vi "parameter error estimate.vi"(8 "covariance":T1, 9 "best fit parameters":dbl[](array[numeric]), 10 "best nonlinear fit":dbl[](array[numeric]), 11 "Y":dbl[](array[numeric])) -> (1 "R-square":dbl, 2 "FWHM":dbl, 3 "Parameters Fit":T2)   [LabVIEW 2023]
uses:
  <vilib>/Analysis/Matrix/Datatypes/RealMatrix.ctl
  <vilib>/Analysis/Matrix/Numeric/Conversions/Array To Matrix - RA2.vi
  <vilib>/Analysis/NI_AALPro.lvlib
  <vilib>/Analysis/Matrix/NI_Matrix.lvlib
panel:
  out "Correlation Matrix":T1
  out "Error":dbl[](array[numeric])
  out "RMSE":dbl
  out "SSE":dbl
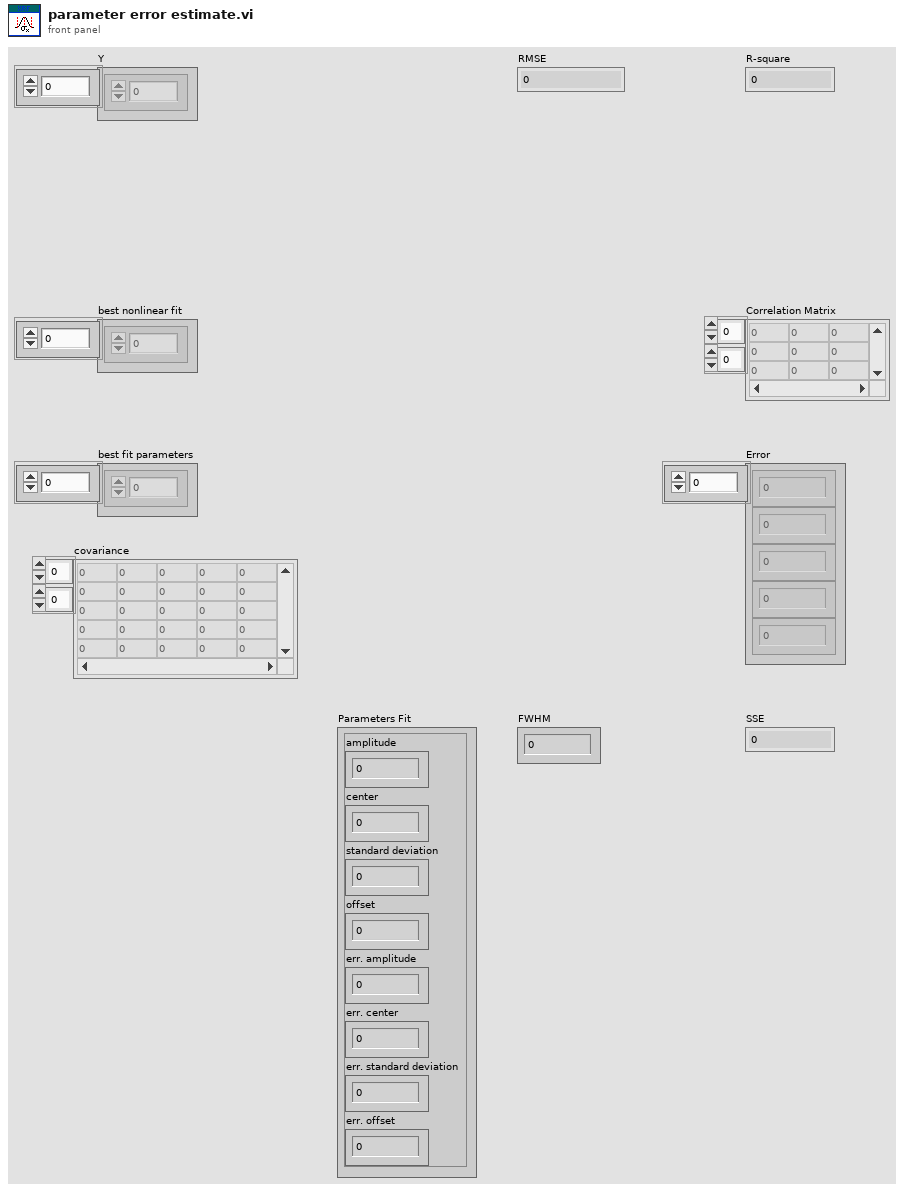
[diagram p1: front panel]
types:
  T1 = typedef "NI_Matrix.lvlib/RealMatrix.ctl" = dbl[][]
  T2 = cluster{"amplitude":dbl, "center":dbl, "standard deviation":dbl, "offset":dbl, "err. amplitude":dbl, "err. center":dbl, "err. standard deviation":dbl, "err. offset":dbl}
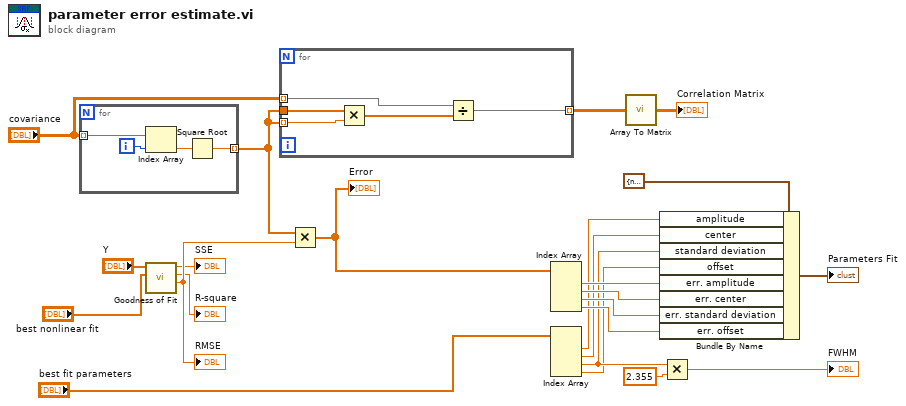
[diagram p0: block diagram]
diagram:
  n1 = for {
    tunnel: "covariance" -> [w27] mode=indexing
    tunnel: [w24] -> w4 mode=indexing
    i -> [w26]
    n2 = Index Array(array=w27, index=w26) -> (element=w25:dbl)
    n3 = Square Root(x=w25) -> (sqrt(x)=w24:dbl)
  }
  n4 = call <vilib>:"Goodness of Fit.vi"("Best Fit"="best nonlinear fit", "Y"="Y") -> ("RMSE"=w22:dbl, "R-square"=→"R-square":dbl, "SSE"=→"SSE":dbl)  [unwired: 6 in, 1 out]
  "RMSE" <- w22
  n5 = for {
    tunnel: "covariance" -> [w29] mode=indexing
    tunnel: w4 -> [w31]
    tunnel: w4 -> [w32] mode=indexing
    tunnel: [w28] -> w5 mode=indexing
    n6 = Multiply(x=w31, y=w32) -> (x*y=w30:dbl[])
    n7 = Divide(x=w29, y=w30) -> (x/y=w28:dbl[])
  }
  n8 = Multiply(x=w4, y=w22) -> (x*y=w21:dbl[])
  "Error" <- w21
  n9 = Index Array(array=w21) -> (element #1=w15:dbl, element #2=w14:dbl, element #3=w13:dbl, element #4=w12:dbl)  [unwired: 4 in]
  n10 = Index Array(array="best fit parameters") -> (element #1=w8:dbl, element #2=w7:dbl, element #3=w10:dbl, element #4=w6:dbl)  [unwired: 4 in]
  n11 = call-poly <vilib>:"Array To Matrix.vi"("Real 2D Array"=w5) -> ("Real Matrix"=→"Correlation Matrix":T1)
  n12 = Bundle By Name(cluster=T2 {"amplitude"=nan, "center"=nan, "standard deviation"=nan, "offset"=nan, "err. amplitude"=nan, "err. center"=nan, "err. standard deviation"=nan, "err. offset"=nan} ("initial guess"), "amplitude"=w8, "center"=w7, "standard deviation"=w10, "offset"=w6, "err. amplitude"=w15, "err. center"=w14, "err. standard deviation"=w13, "err. offset"=w12) -> (→"Parameters Fit":T2)
  n13 = Multiply(x=w10, y=2.355) -> (x*y=→"FWHM":dbl)
